vi "RTD Simulation PointByPoint.vi"() -> ()   [LabVIEW 8.6]
uses:
  vi.lib/UeiDaq/UeiDaqConfigureTimingForSimpleIO.vi
  vi.lib/UeiDaq/UeiDaqReadOneScaledScan.vi
  vi.lib/UeiDaq/UeiDaqWriteOneScaledScan.vi
  vi.lib/UeiDaq/UeiDaqCreateAISession.vi
panel:
  in  "Temperature Scale":i32(ring) items=["Celsius", "Fahrenheit", "Kelvin", "Rankine"]
  in  "Output Values":dbl[](array[numeric])
  in  "AO Resource":string
  out "Waveform Chart":dbl[][](graph)
  in  "Refresh rate (ms)":u32
  in  "stop":bool
  in  "Diag Resource":string
  # "Simulate RTD on RTD-388 and read-back using diagnostic channels"
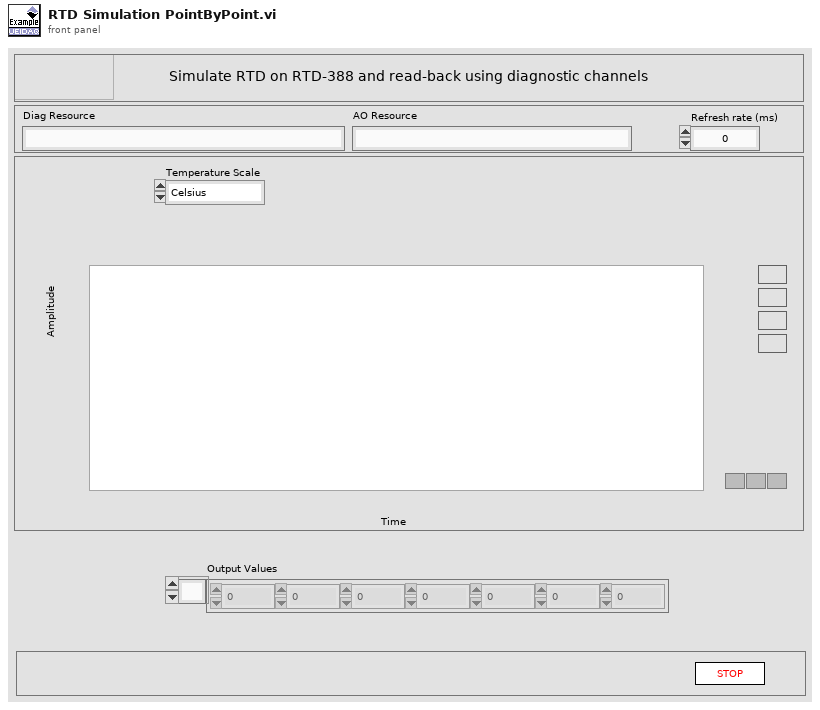
[diagram p1: front panel]
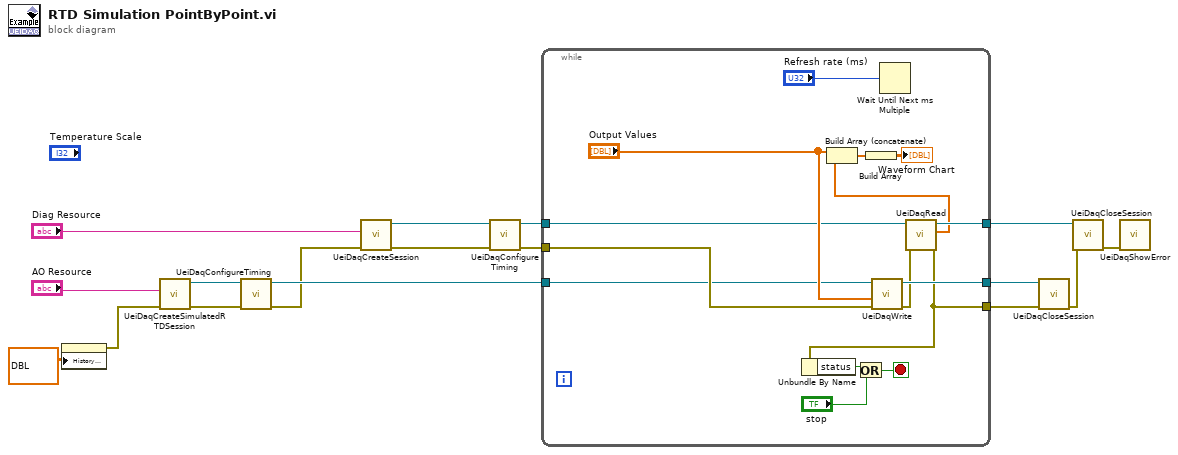
[diagram p0: block diagram]
diagram:
  n1 = property on="Waveform Chart" class="WFChart (strict)"("History Data"=dbl[][] ?) -> (error out=w4:errorcluster)  [unwired: 2 in, 1 out]
  n2 = call "UeiDaqCreateSimulatedRTDSession.vi"("error in (no error)"=w4, "Resource"="AO Resource") -> ("error out"=w15:errorcluster, "UeiDaq Refnum Out"=w16:refnum<k20>)  [unwired: 8 in]
  n3 = call-poly "UeiDaqConfigureTiming.vi"("error in (no error)"=w15, "UeiDaq Refnum In"=w16) -> ("error out"=w10:errorcluster, "UeiDaq Refnum Out"=w14:refnum<k20>)  [unwired: 8 out]
  n4 = call-poly "UeiDaqCreateSession.vi"("error in (no error)"=w10, "Resource"="Diag Resource") -> ("error out"=w2:errorcluster, "UeiDaq Refnum Out"=w3:refnum<k20>)  [unwired: 4 in, 4 out]
  n5 = call-poly "UeiDaqConfigureTiming.vi"("error in (no error)"=w2, "UeiDaq Refnum In"=w3) -> ("error out"=w1:errorcluster, "UeiDaq Refnum Out"=w11:refnum<k20>)  [unwired: 8 out]
  n6 = while {
    tunnel: w14 -> [w19]
    tunnel: [w30] -> w17
    tunnel: w11 -> [w18]
    tunnel: [w28] -> w9
    tunnel: [w23] -> w8
    tunnel: w1 -> [w20]
    stop <- w31 stop-if-true
    n7 = call-poly "UeiDaqWrite.vi"("error in (no error)"=w20, "Scaled Data"="Output Values", "UeiDaq Refnum In"=w19) -> ("error out"=w21:errorcluster, "UeiDaq Refnum Out"=w30:refnum<k20>)  [unwired: 1 in, 6 out]
    n8 = Wait Until Next ms Multiple(millisecond multiple="Refresh rate (ms)") -> ()  [unwired: 1 out]
    n9 = call-poly "UeiDaqRead.vi"("error in (no error)"=w21, "UeiDaq Refnum In"=w18) -> ("error out"=w23:errorcluster, "Scaled Data"=w26:dbl[], "UeiDaq Refnum Out"=w28:refnum<k20>)  [unwired: 7 out]
    n10 = Unbundle By Name(w23) -> ("status"=w27:bool)
    n11 = Build Array (concatenate)("Output Values", w26) -> (w25:dbl[])
    n12 = Or(x=w27, y="stop") -> (x .or. y?=w31:bool)
    n13 = Build Array(w25) -> (→"Waveform Chart":dbl[][])
  }
  n14 = call "UeiDaqCloseSession.vi"("error in (no error)"=w8, "UeiDaq Refnum In"=w17) -> ("error out"=w7:errorcluster)  [unwired: 1 in, 8 out]
  n15 = call "UeiDaqCloseSession.vi"("error in (no error)"=w7, "UeiDaq Refnum In"=w9) -> ("error out"=w6:errorcluster)  [unwired: 1 in, 8 out]
  n16 = call "UeiDaqShowError.vi"("error in (no error)"=w6) -> ()  [unwired: 2 in, 9 out]
